vi "saveTestParameters.vi"(8 "error in (no error)":errorcluster, 11 "Logger in":refnum<class "StiffnessLog.lvclass">) -> (0 "error out":errorcluster, 3 "Logger out":refnum<class "StiffnessLog.lvclass">)   [LabVIEW 2013, in "StiffnessLog.lvclass"]
uses:
  StiffnessLog.lvclass
  <userlib>/Common/Log/Log/Log.lvclass/Log.ctl
  <userlib>/Common/Log/Log/Log.lvclass
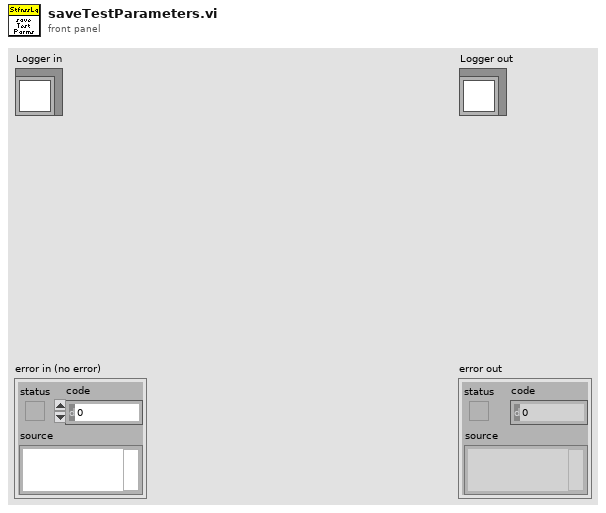
[diagram p1: front panel]
types:
  T1 = typedef "Log.lvlib/Log.ctl" = cluster{"Log Directory":path, "Log Filename Base":string, "Max records per file":u32, "Comment":string}
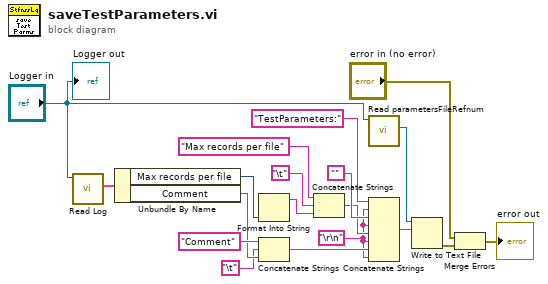
[diagram p0: block diagram]
diagram:
  w5 = "\r\n"
  n1 = call <userlib>:"Read Log.vi"("Log in"="Logger in") -> ("Log"=w19:T1)  [unwired: 9 in, 1 out]
  n2 = Unbundle By Name(w19) -> ("Max records per file"=w18:u32, "Comment"=w8:string)
  n3 = Format Into String(w18) -> (resulting string=w11:string)  [unwired: 3 in, 1 out]
  n4 = Concatenate Strings("Comment" ("element"), "\t", w8) -> (w6:string)
  n5 = Concatenate Strings("Max records per file" ("element"), "\t", w11) -> (w10:string)
  n6 = call <userlib>:"Read parametersFileRefnum.vi"("Log in"="Logger in") -> ("parametersFileRefnum"=w16:refnum<file>)  [unwired: 9 in, 1 out]
  n7 = Concatenate Strings("TestParameters:", w5, "", w5, w10, w5, w6, w5) -> (w4:string)
  n8 = Write to Text File(file (use dialog)=w16, text=w4) -> (error out=w3:errorcluster)  [unwired: 2 in, 2 out]
  n9 = Merge Errors("error in (no error)", w3) -> (→"error out":errorcluster)
  "Logger out" <- "Logger in"
